vi "subfft.vi"(2 "y-signal":dbl[](array[numeric]) format="%.2f", 3 "time step":dbl format="%.2f") -> (0 "Phase":cluster{"f0":dbl, "df":dbl, "real part":dbl[]} {"real part" format="%.2f"; "df" format="%.2f"; "f0" format="%.2f"}, 1 "Amplitude":cluster{"f0":dbl, "df":dbl, "real part":dbl[]} {"real part" format="%.2f"; "df" format="%.2f"; "f0" format="%.2f"})   [LabVIEW 2010]
uses:
  <vilib>/measure/maspectr.llb/FFT Spectrum (Mag-Phase) for 1 Chan.vi
  <vilib>/measure/NI_MAPro.lvlib
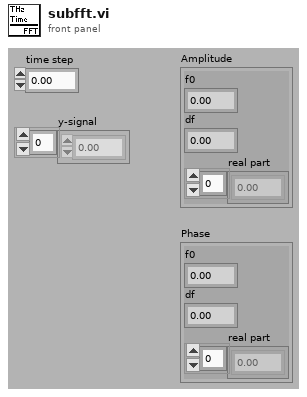
[diagram p1: front panel]
types:
  T1 = cluster{"dB On (F)":bool, "unwrap phase (F)":bool, "convert to degree (F)":bool}
  T2 = enum16{"None ", "Hanning", "Hamming", "Blackman-Harris", "Exact Blackman", "Blackman", "Flat Top", "4 Term B-Harris ", "7 Term B-Harris", "Low Sidelobe"}
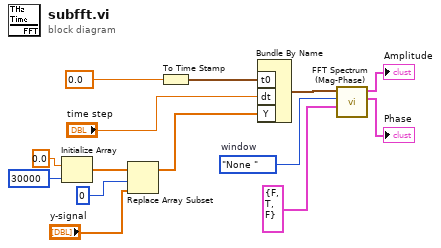
[diagram p0: block diagram]
diagram:
  w9 = T2."None "  # window
  n1 = Initialize Array(0.0 ("원소"), 30000 ("차원 크기")) -> (w5:dbl[])
  n2 = Replace Array Subset(array=w5, new element="y-signal", index=0 ("인덱스")) -> (w2:dbl[])
  n3 = To Time Stamp(1:0.0 ("t0")) -> (0:w8:timestamp)
  n4 = Bundle By Name("t0"=w8, "dt"="time step", "Y"=w2) -> (w11:waveform(dbl))  [unwired: 1 in]
  n5 = call-poly <vilib>:"FFT Spectrum (Mag-Phase).vi"("view"=T1 {"dB On (F)"=FALSE, "unwrap phase (F)"=TRUE, "convert to degree (F)"=FALSE}, "window"=w9, "time signal"=w11) -> ("phase"=→"Phase":cluster{"f0":dbl, "df":dbl, "phase":dbl[]}, "magnitude"=→"Amplitude":cluster{"f0":dbl, "df":dbl, "magnitude":dbl[]})  [unwired: 4 in, 3 out]
